vi "ParseFileName.vi"(0 "String in":string) -> (1 "Info":cluster{"Set":string, "Position":i32, "Tap":i32}, 2 "Name":T1, 3 "Everything else":string)   [LabVIEW 2022 SP3]
uses:
  <vilib>/Utility/error.llb/Trim Whitespace One-Sided.vi
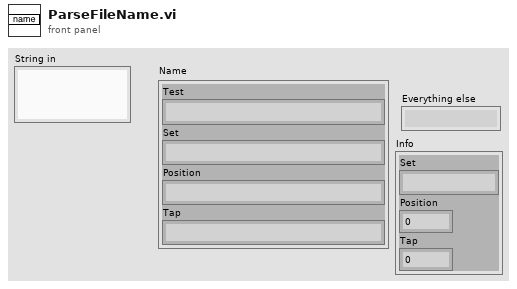
[diagram p1: front panel]
types:
  T1 = cluster{"Test":string, "Set":string, "Position":string, "Tap":string}
  T2 = cluster{"Instrument":string, "Set":string, "Position":string, "Tap":string}
  T3 = cluster{"trimmed string":string, "trimmed string":string, "trimmed string":string, "trimmed string":string}
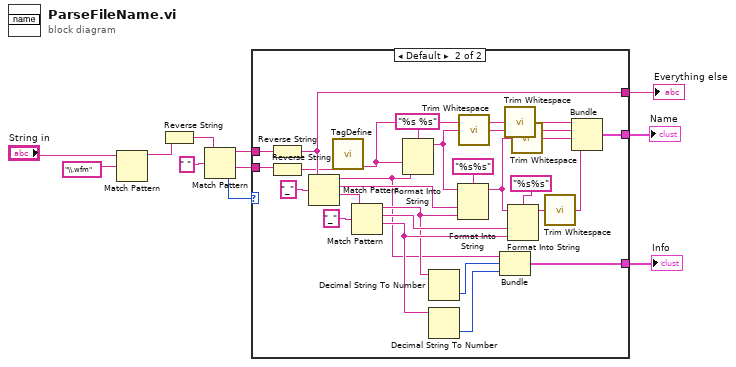
[diagram p0: block diagram]
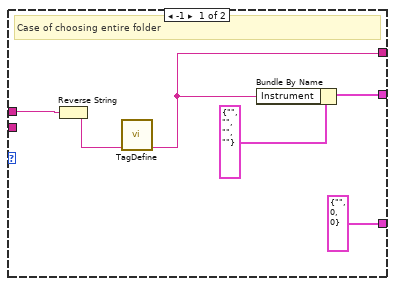
[diagram p2: hidden frame]
diagram:
  n1 = Match Pattern(string="String in", regular expression="\\.wfm") -> (before substring=w1:string)  [unwired: 1 in, 3 out]
  n2 = Reverse String(1:w1) -> (0:w2:string)
  n3 = Match Pattern(string=w2, regular expression=" ") -> (before substring=w11:string, after substring=w9:string, offset past match=w5:i32)  [unwired: 1 in, 1 out]
  n4 = case shown="Default" w5 {
    tunnel: w11 -> [w17 w44]
    tunnel: w9 -> [_ w43]
    tunnel: [w12 w36] -> w8
    tunnel: [w15 w30] -> w7
    tunnel: [cluster{string, i32, i32} {"", 0, 0} w24] -> w6
    frame -1 {
      # "Case of choosing entire folder"
      n5 = Reverse String(1:w17) -> (0:w13:string)
      n6 = call "TagDefine.vi"("LUT in"=w13) -> ("String Out"=w12:string)  [unwired: 9 in, 1 out]
      n7 = Bundle By Name(cluster=T2 {"Instrument"="", "Set"="", "Position"="", "Tap"=""} ("Name"), "Instrument"=w12) -> (w15:T2)
    }
    frame Default {
      n8 = Reverse String(1:w44) -> (0:w36:string)
      n9 = Reverse String(1:w43) -> (0:w23:string)
      n10 = Match Pattern(string=w36, regular expression="_") -> (before substring=w27:string, match substring=w35:string, after substring=w37:string)  [unwired: 1 in, 1 out]
      n11 = call "TagDefine.vi"("LUT in"=w23) -> ("String Out"=w22:string)  [unwired: 9 in, 1 out]
      n12 = Match Pattern(string=w37, regular expression="_") -> (before substring=w28:string, match substring=w34:string, after substring=w29:string)  [unwired: 1 in, 1 out]
      n13 = Format Into String(format string="%s %s", w22, w27) -> (resulting string=w33:string)  [unwired: 2 in, 1 out]
      n14 = Decimal String To Number(string=w28) -> (number=w26:i32)  [unwired: 2 in, 1 out]
      n15 = Decimal String To Number(string=w29) -> (number=w25:i32)  [unwired: 2 in, 1 out]
      n16 = Format Into String(format string="%s%s", initial string=w33, w35, w28) -> (resulting string=w32:string)  [unwired: 1 in, 1 out]
      n17 = call <vilib>:"Trim Whitespace.vi"("string"=w33) -> ("trimmed string"=w20:string)  [unwired: 1 in]
      n18 = Bundle(w27, w26, w25) -> (w24:cluster{string, i32, i32})  [unwired: 1 in]
      n19 = call <vilib>:"Trim Whitespace.vi"("string"=w22) -> ("trimmed string"=w21:string)  [unwired: 1 in]
      n20 = Format Into String(format string="%s%s", initial string=w32, w34, w29) -> (resulting string=w31:string)  [unwired: 1 in, 1 out]
      n21 = call <vilib>:"Trim Whitespace.vi"("string"=w32) -> ("trimmed string"=w19:string)  [unwired: 1 in]
      n22 = call <vilib>:"Trim Whitespace.vi"("string"=w31) -> ("trimmed string"=w18:string)  [unwired: 1 in]
      n23 = Bundle("trimmed string"=w21, "trimmed string"=w20, "trimmed string"=w19, "trimmed string"=w18) -> (w30:T3)  [unwired: 1 in]
    }
  }
  "Everything else" <- w8
  "Name" <- w7
  "Info" <- w6
